vi "calc_focus.vi"(8 "error in":errorcluster, 11 "Image":T1) -> (0 "error out":errorcluster, 2 "focus":sgl, 3 "Image out":T1)   [LabVIEW 2024, in "Vision.lvlib"]
uses:
  Vision.lvlib
  <vilib>/vision/Image Controls.llb/IMAQ Image.ctl
  bin/PatternRecognition.dll
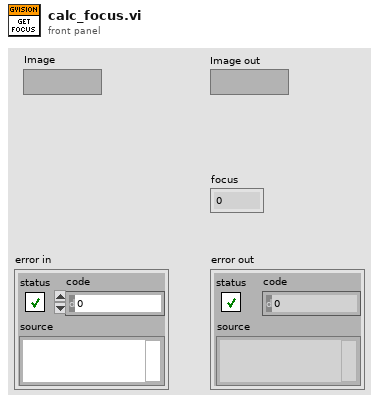
[diagram p1: front panel]
types:
  T1 = typedef "IMAQ Image.ctl" = refnum<image>
  T2 = enum32{"Map Pixel Pointer", "Unmap Pixel Pointer", "Get Pixels Infos"}
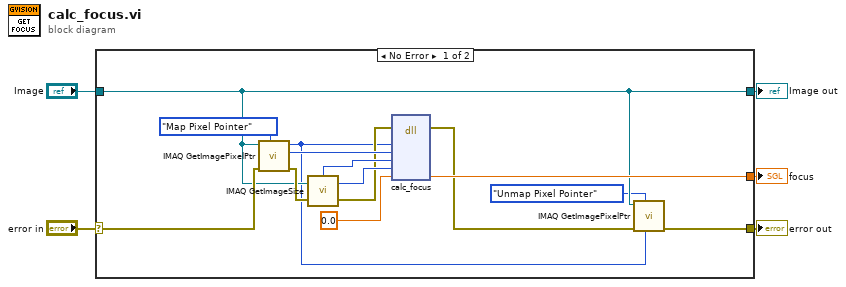
[diagram p0: block diagram]
diagram:
  n1 = case shown="No Error" "error in" {
    selector: "error in" -> [w11 w21]
    tunnel: [w6 w21] -> w5
    tunnel: [w19 _] -> w4
    tunnel: "Image" -> [w10 w20]
    tunnel: [w10 w20] -> w1
    frame No Error {
      n2 = call "IMAQ GetImagePixelPtr"("Function"=T2."Map Pixel Pointer", "error in (no error)"=w11, "Image"=w10) -> ("error out"=w16:errorcluster, "LineWidth(Pixels)"=w15:i32, "Pixel Pointer out"=w7:u64)  [unwired: 3 in, 3 out]
      n3 = call "IMAQ GetImageSize"("Image"=w10, "error in (no error)"=w16) -> ("Y Resolution"=w13:i32, "X Resolution"=w14:i32, "error out"=w12:errorcluster)  [unwired: 2 in]
      n4 = dll-call lib="C:/Users/cfang/Desktop/nebraska-silicon-lab/pixel-gantry-control/Gantry/Shared Components/bin/PatternRecognition.dll" fn="calc_focus"(error in=w12, "img"=w7, "imgLineWidth"=w15, "imgWidth"=w14, "imgHeight"=w13, "focus"=sgl 0.0) -> (error out=w9:errorcluster, "focus"=w19:sgl)  [unwired: 7 in, 1 out]
      n5 = call "IMAQ GetImagePixelPtr"("Pixel Pointer in"=w7, "Function"=T2."Unmap Pixel Pointer", "error in (no error)"=w9, "Image"=w10) -> ("error out"=w6:errorcluster)  [unwired: 2 in, 5 out]
    }
    frame Error {
    }
  }
  "error out" <- w5
  "focus" <- w4
  "Image out" <- w1
